vi "FM_RTL-SDR_RX_atan2_VI.vi"() -> (3 "Calculation Time (s)":dbl)   [LabVIEW 2013]
doc: "Demonstrates how to use the MATLAB script node. The m-file script is used to calculate the data and the resulting fractal is displayed on the front panel. The MathWorks, Inc. MATLAB (R) Application Software version 5.0 or later must be installed and properly licensed in order to run this VI."
uses:
  <vilib>/Waveform/WDTFileIO.llb/Read Waveform from File.vi
  <vilib>/Analysis/NI_AALPro.lvlib
panel:
  out "Baseband":dbl[](array[numeric])
  in  "file path":path=path "D:/File/Recoder_Data_IQIQ"
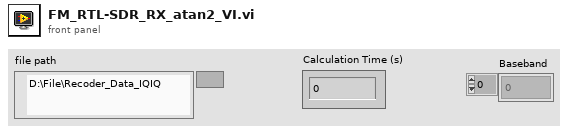
[diagram p1: front panel]
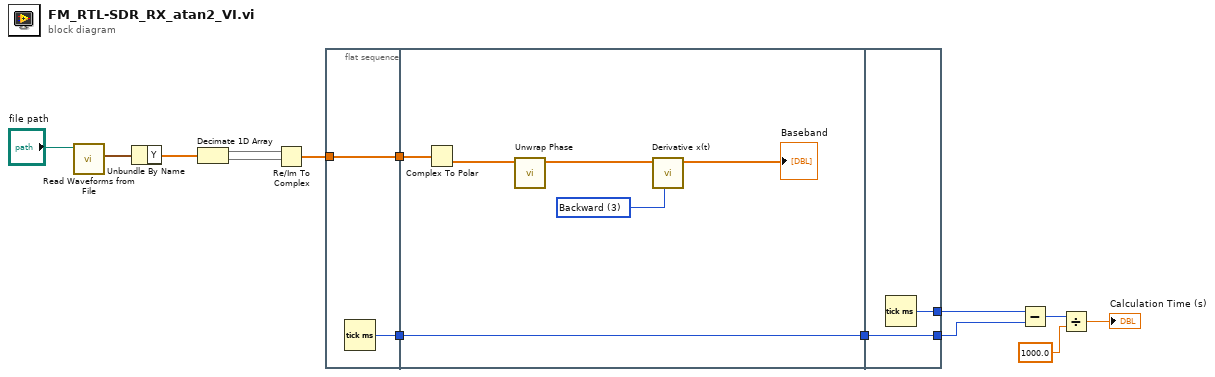
[diagram p0: block diagram]
diagram:
  n1 = call-poly <vilib>:"Read Waveforms from File.vi"("file path (dialog if empty)"="file path") -> ("first waveform in record"=w7:waveform(dbl))  [unwired: 5 in, 3 out]
  n2 = Unbundle By Name(w7) -> ("Y"=w5:dbl[])
  n3 = Decimate 1D Array(w5) -> (w4:dbl[], w3:dbl[])
  n4 = Re/Im To Complex(1:w3, 2:w4) -> (0:w2:cdb[])
  n5 = flat-sequence {
    tunnel: [w16] -> w8
    tunnel: w2 -> [w15]
    tunnel: [w15] -> w1
    tunnel: [w22] -> w14
    tunnel: w8 -> [w22]
    tunnel: w1 -> [w18]
    tunnel: w14 -> [w23]
    tunnel: [w24] -> w11
    tunnel: [w23] -> w10
    frame #0 {
      n6 = Tick Count (ms)() -> (millisecond timer value=w16:u32)
    }
    frame #1 {
      w19 = u16 3 items=["2nd Order Central", "4th Order Central", "Forward", "Backward"] ("method")
      n7 = Complex To Polar(r * e^(i*theta)=w18) -> (theta=w21:dbl[])  [unwired: 1 out]
      n8 = call <vilib>:"Unwrap Phase.vi"("Phase"=w21) -> ("Unwrapped Phase"=w20:dbl[])  [unwired: 9 in, 1 out]
      n9 = call <vilib>:"Derivative x(t).vi"("method"=w19, "X"=w20) -> ("dX/dt"=→"Baseband":dbl[])  [unwired: 8 in, 1 out]
    }
    frame #2 {
      n10 = Tick Count (ms)() -> (millisecond timer value=w24:u32)
    }
  }
  n11 = Subtract(x=w11, y=w10) -> (x-y=w12:u32)
  n12 = Divide(x=w12, y=1000.0) -> (x/y=→"Calculation Time (s)":dbl)
